vi "ex9-4.vi"() -> ()   [LabVIEW 2009]
uses:
  <vilib>/NXT/Subs/MotorOutput.ctl
  <vilib>/Utility/inputDevices.llb/closeJoystick.vi
  <vilib>/Utility/inputDevices.llb/joystickAcquire.vi
panel:
  out "右馬達電力":dbl(slide) scale=-100.0..100.0
  out "左馬達電力":dbl(slide) scale=-100.0..100.0
  out "方向資訊":T1
  out "軸向資訊":T2
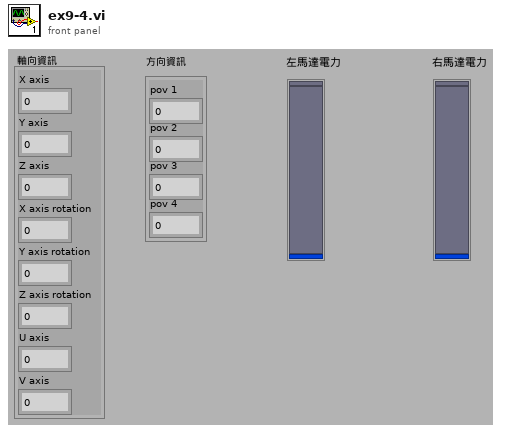
[diagram p1: front panel]
types:
  T1 = cluster{"pov 1":i32, "pov 2":i32, "pov 3":i32, "pov 4":i32}
  T2 = cluster{"X axis":i32, "Y axis":i32, "Z axis":i32, "X axis rotation":i32, "Y axis rotation":i32, "Z axis rotation":i32, "U axis":i32, "V axis":i32}
  T3 = typedef "MotorOutput.ctl" = u8
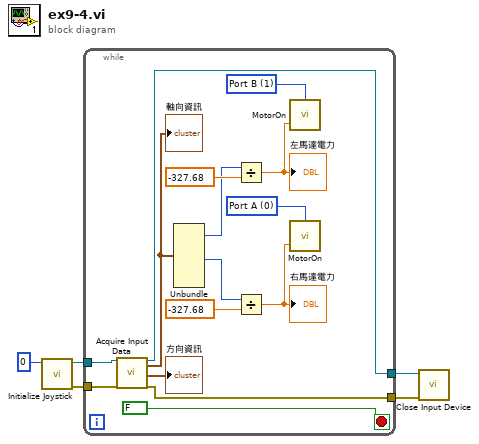
[diagram p0: block diagram]
diagram:
  n1 = call <vilib>:"Initialize Joystick.vi"("device index"=0) -> ("error out"=w4:errorcluster, "device ID"=w5:refnum<k1>)  [unwired: 9 in]
  n2 = while {
    tunnel: w5 -> [w20]
    tunnel: w4 -> [w19]
    tunnel: [w18] -> w3
    tunnel: [w17] -> w2
    stop <- FALSE stop-if-true
    w14 = T3 1 items=["Port A", "Port B", "Port C", "All Ports"] ("Output Port (All Ports)")
    w13 = T3 0 items=["Port A", "Port B", "Port C", "All Ports"] ("Output Port (All Ports)")
    n3 = call-poly <vilib>:"Acquire Input Data.vi"("device ID"=w20, "error in (no error)"=w19) -> ("device ID"=w18:refnum<k1>, "axis info"=w16:T2, "direction info"=→"方向資訊":T1, "error out"=w17:errorcluster)  [unwired: 13 in, 1 out]
    "軸向資訊" <- w16
    n4 = Unbundle(w16) -> ("Y axis"=w11:i32, "Y axis rotation"=w8:i32)  [unwired: 6 out]
    n5 = Divide(x=w11, y=-327.68) -> (x/y=w7:dbl)
    "左馬達電力" <- w7
    n6 = Divide(x=w8, y=-327.68) -> (x/y=w6:dbl)
    "右馬達電力" <- w6
    n7 = call <vilib>:"MotorOn.vi"("Power (75)"=w7, "Output Port (All Ports)"=w14) -> ()  [unwired: 2 in, 1 out]
    n8 = call <vilib>:"MotorOn.vi"("Power (75)"=w6, "Output Port (All Ports)"=w13) -> ()  [unwired: 2 in, 1 out]
  }
  n9 = call-poly <vilib>:"Close Input Device.vi"("error in (no error)"=w2, "device ID"=w3) -> ()  [unwired: 8 in, 1 out]
